vi "Previous Available Datum Index.vi"(1 "bytestream":refnum<class "Bytestream.lvclass">) -> (0 "index":i32)   [LabVIEW 2020, in "NI_Bytestream.lvlib" / "Bytestream.lvclass"]
uses:
  <vilib>/Array/Bytestream/Bytestream.lvclass
  <vilib>/Array/Bytestream/Bytestream.lvclass/Bytestream.ctl
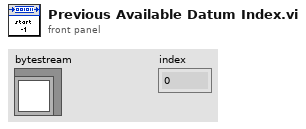
[diagram p1: front panel]
types:
  T1 = typedef "NI_Bytestream.lvlib/Bytestream.lvclass/Datum.ctl" = cluster{"array":u8[], "index":i32}
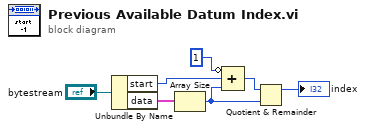
[diagram p0: block diagram]
diagram:
  n1 = Unbundle By Name("bytestream") -> ("start"=w4:i32, "data"=w6:T1[])
  n2 = Array Size(array=w6) -> (size(s)=w3:i32)
  n3 = Compound Arithmetic op=ADD(invert 1 ("value"), w4, w3) -> (w1:i32)
  n4 = Quotient & Remainder(x=w1, y=w3) -> (x-y*floor(x/y)=→"index":i32)  [unwired: 1 out]
